vi "Find (array).vi"(8 "error in (no error)":errorcluster, 11 "Parameter to Hardware Map in":refnum<class "Parameter to Hardware Map.lvclass">) -> (0 "error out":errorcluster, 3 "Parameter to Hardware Map out":refnum<class "Parameter to Hardware Map.lvclass">)   [LabVIEW 2020, in "RxnRover.lvlib" / "Parameter to Hardware Map.lvclass"]
doc: "Find the elements from the map matching the given keys. A parallel boolean array is provided, where each entry indicates whether the key-value pair in the corresponding Key-Value Pairs output array position was found.s"
uses:
  Parameter to Hardware Map.lvclass
  Pair.ctl
  Controller/Generic Plugin.lvclass
panel:
  out "Found?":bool[](array[boolean])
  out "Key-Value Pairs":T1[](array[typedef])
  in  "Keys":string[](array[string])
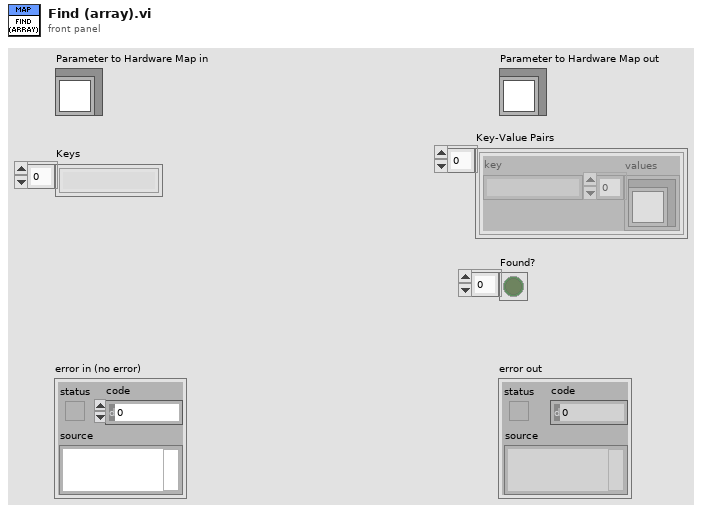
[diagram p1: front panel]
types:
  T1 = typedef "RxnRover.lvlib/Parameter to Hardware Map.lvclass/Pair.ctl" = cluster{"key":string, "values":refnum<class "Generic Plugin.lvclass">[]}
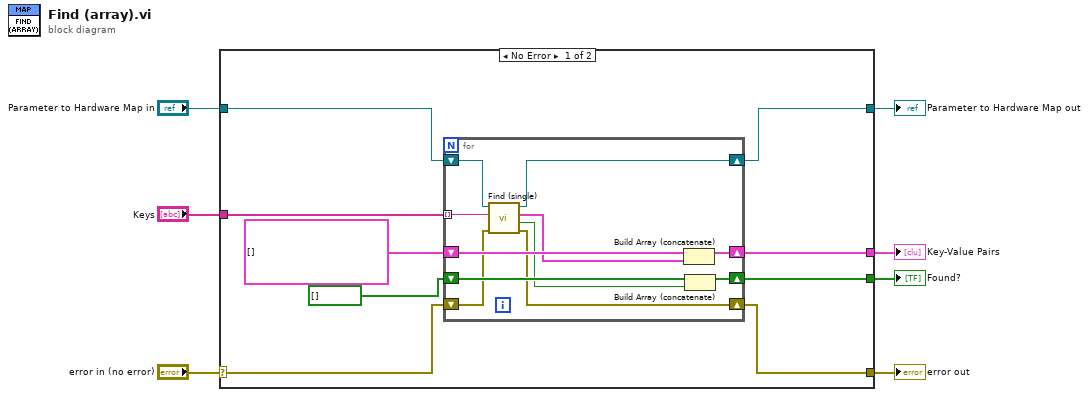
[diagram p0: block diagram]
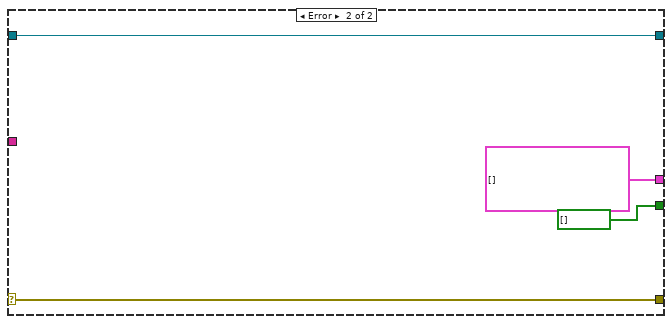
[diagram p2: hidden frame]
diagram:
  n1 = case shown="No Error" "error in (no error)" {
    selector: "error in (no error)" -> [w14 w31]
    tunnel: [w13 w31] -> w6
    tunnel: [w15 w30] -> w4
    tunnel: "Parameter to Hardware Map in" -> [w16 w30]
    tunnel: "Keys" -> [w12 _]
    tunnel: [w9 bool[] []] -> w2
    tunnel: [w8 T1[] [] ("Key-Value Pairs")] -> w1
    frame No Error {
      n2 = for {
        shift-right: [w19] -> w15
        shift-left: w16 -> [w20]
        shift-right: [w17] -> w13
        shift-left: w14 -> [w18]
        tunnel: w12 -> [w27] mode=indexing
        shift-right: [w25] -> w8
        shift-left: T1[] [] ("Key-Value Pairs") -> [w26]
        shift-right: [w21] -> w9
        shift-left: bool[] [] -> [w23]
        n3 = call "Find (single).vi"("error in (no error)"=w18, "Key"=w27, "Parameter to Hardware Map in"=w20) -> ("error out"=w17:errorcluster, "Found?"=w22:bool, "Key-Value Pair"=w24:T1, "Parameter to Hardware Map out"=w19:refnum<class "Parameter to Hardware Map.lvclass">)  [unwired: 5 in]
        n4 = Build Array (concatenate)(w26, w24) -> (w25:T1[])
        n5 = Build Array (concatenate)(w23, w22) -> (w21:bool[])
      }
    }
    frame Error {
    }
  }
  "error out" <- w6
  "Parameter to Hardware Map out" <- w4
  "Found?" <- w2
  "Key-Value Pairs" <- w1
